vi "TestApp.vi"   [LabVIEW 2021]
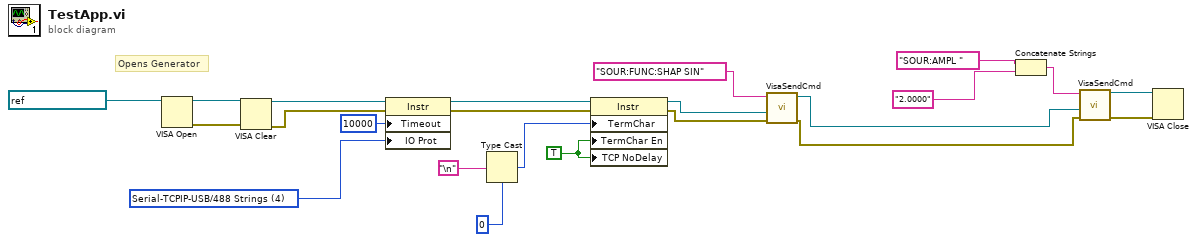
[diagram p0: block diagram]
diagram:
  w14 = TRUE
  w18 = u16 4 items=["Normal"=1, "VXI/FDC"=2, "GPIB/HS488"=3, "Serial-TCPIP-USB/488 Strings"=4, "USBTMC/Vendor-Specific"=5] ("Message Based Settings:IO Protocol")
  # "Opens Generator"
  n1 = VISA Open(VISA resource name=refnum<visa-resource-name> "FG_Simulator") -> (VISA resource name=w12:refnum<visa-resource-name>, error out=w11:errorcluster)  [unwired: 4 in]
  n2 = VISA Clear(VISA resource name=w12, error in (no error)=w11) -> (VISA resource name out=w23:refnum<visa-resource-name>, error out=w22:errorcluster)
  n3 = property class="Instr"(reference=w23, error in=w22, "Timeout"=u32 10000 ("General Settings:Timeout Value"), "IO Prot"=w18) -> (reference out=w21:refnum<visa-resource-name>, error out=w20:errorcluster)
  n4 = Type Cast(type=0, x="\n") -> (*(type *) &x=w15:i32)
  n5 = property class="Instr"(reference=w21, error in=w20, "TermChar"=w15, "TermChar En"=w14, "TCP NoDelay"=w14) -> (reference out=w9:refnum<visa-resource-name>, error out=w8:errorcluster)
  n6 = call "VisaSendCmd.vi"("error in (no error)"=w8, "VISA resource name"=w9, "Msg to send"="SOUR:FUNC:SHAP SIN") -> ("error out"=w4:errorcluster, "VISA resource output"=w5:refnum<visa-resource-name>)  [unwired: 7 in]
  n7 = Concatenate Strings("SOUR:AMPL ", "2.0000" ("string")) -> (w6:string)
  n8 = call "VisaSendCmd.vi"("error in (no error)"=w4, "VISA resource name"=w5, "Msg to send"=w6) -> ("error out"=w1:errorcluster, "VISA resource output"=w2:refnum<visa-resource-name>)  [unwired: 7 in]
  n9 = VISA Close(VISA resource name=w2, error in (no error)=w1) -> ()  [unwired: 1 out]
